vi "SS_Delay_Duration.vi"(6 "Main Cluster IN":T1, 7 "Scan Rate (ms)":i32, 8 "Error In":errorcluster, 11 "Info In":string="\nWaiting for TimerScope Trigger\n- IN: SS TimerScope Trigger\n- OUT: SET SS ThermoRec Received Trigger\nPulse Number is 231123\nPulse Type is 4\n\nDuration (s) is  2.000000\nDelay (s)  is  1.000000\nScan Period (ms) is  15\nNumber of Samples is  134\n\nDelay Started\nDelay Complete\nExternal Measurement of Delay (s): 1.000000\nACQUIRING DATA") -> (0 "Error Out":errorcluster, 3 "Info Out":string="\nWaiting for TimerScope Trigger\n- IN: SS TimerScope Trigger\n- OUT: SET SS ThermoRec Received Trigger\nPulse Number is 231123\nPulse Type is 4\n\nDuration (s) is  2.000000\nDelay (s)  is  1.000000\nScan Period (ms) is  15\nNumber of Samples is  134\n\nDelay Started\nDelay Complete\nExternal Measurement of Delay (s): 1.000000\nACQUIRING DATA", 4 "Main Cluster OUT":T1)   [LabVIEW 2016]
uses:
  Control/Control_Main.ctl
  Control/Control_ModuleArray.ctl
panel:
  in  "Tab Control":enum32{"IN", "OUT", "SubVI Info"}(tab)
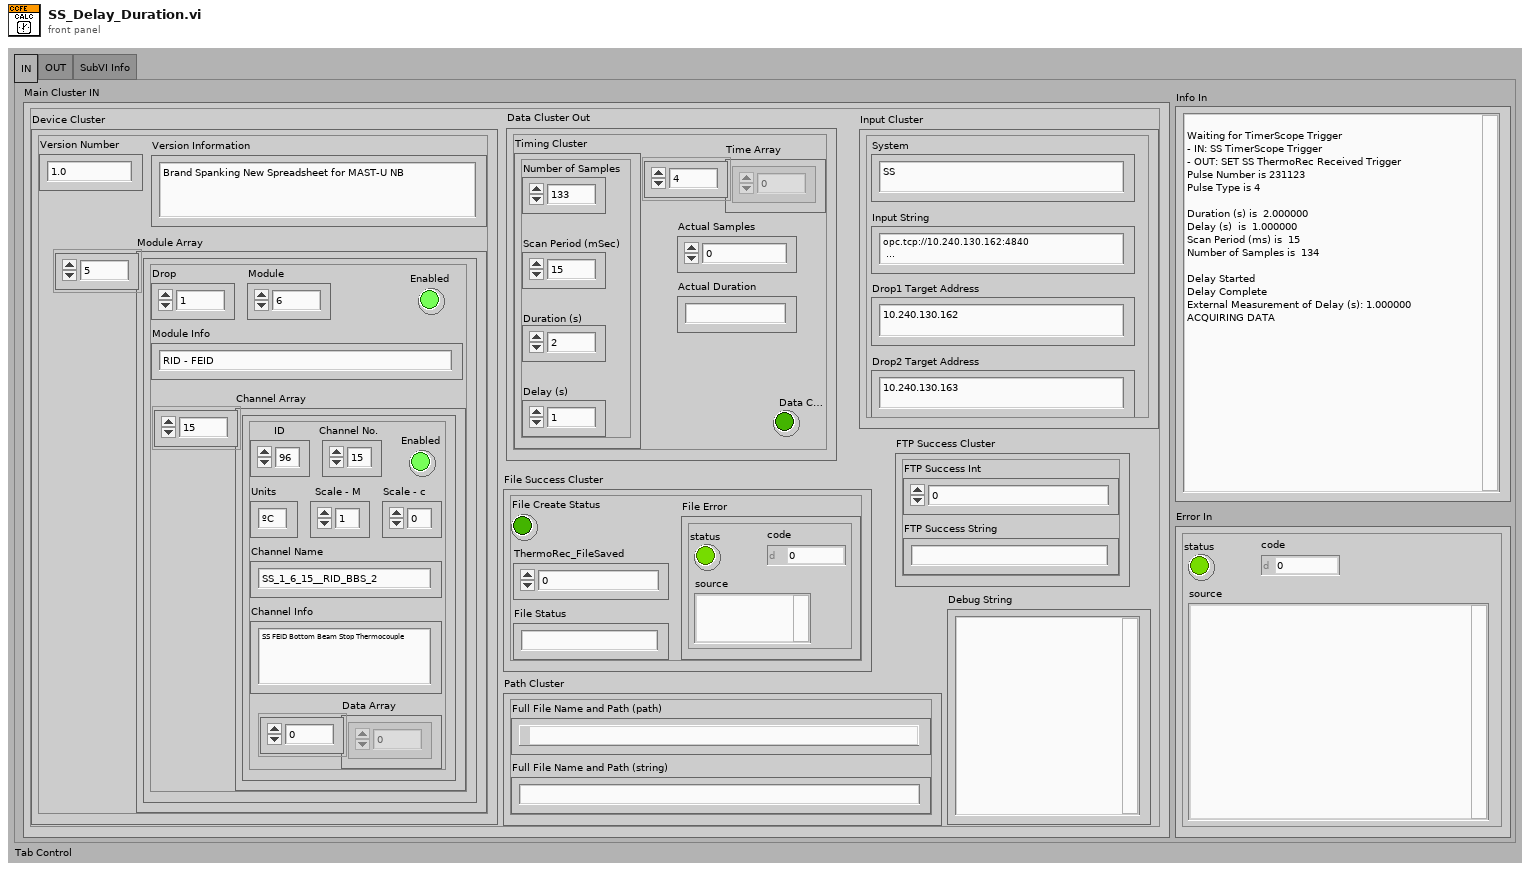
[diagram p1: front panel]
types:
  T1 = typedef "Control_Main.ctl" = cluster{"Device Cluster":cluster{"Module Array":T2, "Version Number":string, "Version Information":string}, "Input Cluster":cluster{"Input String":string, "Drop1 Target Address":string, "Drop2 Target Address":string, "System":string}, "Data Cluster Out":cluster{"Timing Cluster":cluster{"Number of Samples":i32, "Scan Period (mSec)":u32, "Duration (s)":dbl, "Delay (s)":dbl}, "Time Array":dbl[], "Actual Samples":i32, "Actual Duration":string, "Data Collection Error":bool}, "Path Cluster":cluster{"Full File Name and Path (path)":path, "Full File Name and Path (string)":string}, "File Success Cluster":cluster{"ThermoRec_FileSaved":i32, "File Create Status":bool, "File Error":errorcluster, "File Status":string}, "FTP Success Cluster":cluster{"FTP Success Int":i32, "FTP Success String":string}, "Debug String":string}
  T2 = typedef "Control_ModuleArray.ctl" = cluster{"Drop":i32, "Module":i32, "Module Info":string, "Enabled":bool, "Channel Array":cluster{"ID":i32, "Channel No.":i32, "Enabled":bool, "Channel Name":string, "Channel Info":string, "Units":string, "Scale - M":dbl, "Scale - c":dbl, "Data Array":dbl[]}[]}[]
  T3 = cluster{"Number of Samples":i32, "Scan Period (mSec)":u32, "Duration (s)":dbl, "Delay (s)":dbl}
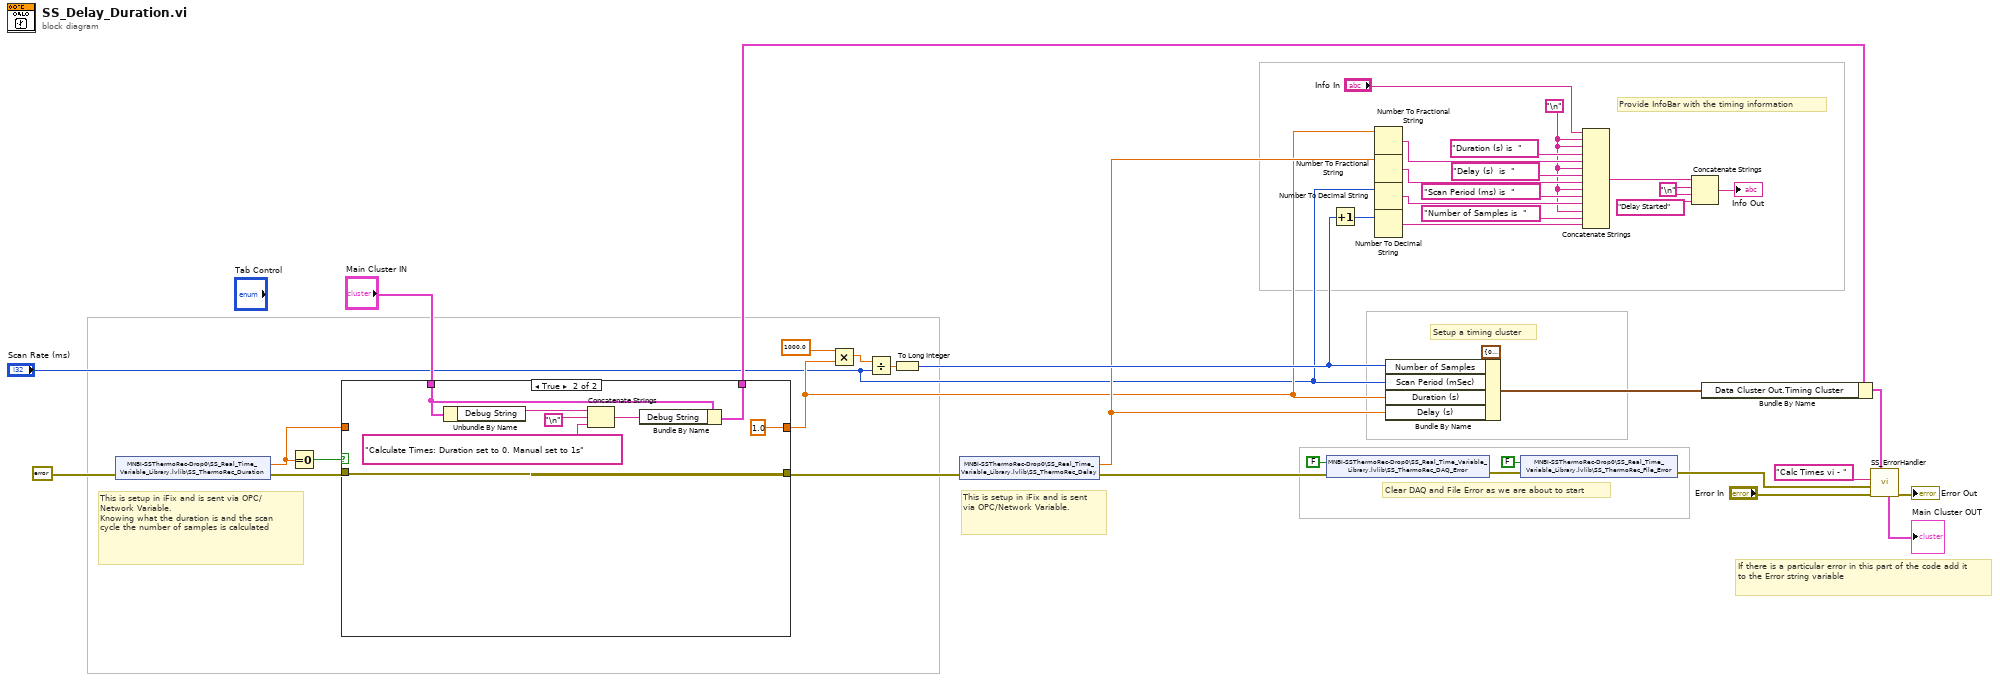
[diagram p0: block diagram]
diagram:
  w27 = "\n"
  w30 = "\n"
  # "This is setup in iFix and is sent via OPC/Network Variable."
  # "If there is a particular error in this part of the code add it to the Error string variable"
  # "Clear DAQ and File Error as we are about to start"
  # "Provide InfoBar with the timing information"
  # "Setup a timing cluster"
  # "This is setup in iFix and is sent via OPC/Network Variable.\nKnowing what the duration is and the scan cycle the number of samples is calculated"
  n1 = shared-variable "MNBI-SSThermoRec-Drop0\\SS_Real_Time_Variable_Library.lvlib\\SS_ThermoRec_Duration"(error in=errorcluster {"status"=FALSE, "code"=0, "source"=""} ("error constant")) -> (w18:dbl, error out=w19:errorcluster)
  n2 = Equal To 0?(x=w18) -> (x = 0?=w20:bool)
  n3 = case shown="True" w20 {
    tunnel: w19 -> [w44 w46]
    tunnel: [w44 w46] -> w16
    tunnel: w18 -> [w43 _]
    tunnel: [w43 1.0 ("y")] -> w7
    tunnel: "Main Cluster IN" -> [w42 w48]
    tunnel: [w42 w49] -> w3
    frame False {
    }
    frame True {
      n4 = Unbundle By Name(w48) -> ("Debug String"=w47:string)
      n5 = Concatenate Strings(w47, "\n", "Calculate Times: Duration set to 0. Manual set to 1s" ("source")) -> (w45:string)
      n6 = Bundle By Name(cluster=w48, "Debug String"=w45) -> (w49:T1)
    }
  }
  n7 = Multiply(x=1000.0, y=w7) -> (x*y=w5:dbl)
  n8 = Divide(x=w5, y="Scan Rate (ms)") -> (x/y=w41:dbl)
  n9 = To Long Integer(number=w41) -> (32bit integer=w32:i32)
  n10 = shared-variable "MNBI-SSThermoRec-Drop0\\SS_Real_Time_Variable_Library.lvlib\\SS_ThermoRec_Delay"(error in=w16) -> (w17:dbl, error out=w15:errorcluster)
  n11 = shared-variable "MNBI-SSThermoRec-Drop0\\SS_Real_Time_Variable_Library.lvlib\\SS_ThermoRec_DAQ_Error"(FALSE ("SS_ThermoRec_DAQ_Error"), error in=w15) -> (error out=w23:errorcluster)
  n12 = Increment(x=w32) -> (x+1=w29:i32)
  n13 = Number To Fractional String(number=w7) -> (F-format string=w39:string)  [unwired: 3 in]
  n14 = Number To Fractional String(number=w17) -> (F-format string=w37:string)  [unwired: 3 in]
  n15 = Number To Decimal String(number="Scan Rate (ms)") -> (decimal integer string=w33:string)  [unwired: 1 in]
  n16 = Number To Decimal String(number=w29) -> (decimal integer string=w31:string)  [unwired: 1 in]
  n17 = Bundle By Name(cluster=T3 {"Number of Samples"=0, "Scan Period (mSec)"=14, "Duration (s)"=0.0, "Delay (s)"=0.0} ("Data Cluster 2"), "Number of Samples"=w32, "Scan Period (mSec)"="Scan Rate (ms)", "Duration (s)"=w7, "Delay (s)"=w17) -> (w22:T3)
  n18 = shared-variable "MNBI-SSThermoRec-Drop0\\SS_Real_Time_Variable_Library.lvlib\\SS_ThermoRec_File_Error"(FALSE ("SS_ThermoRec_DAQ_Error"), error in=w23) -> (error out=w10:errorcluster)
  n19 = Concatenate Strings("Info In", w30, w30, "Duration (s) is  ", w39, w30, "Delay (s)  is  ", w37, w30, "Scan Period (ms) is  ", w33, w30, "Number of Samples is  ", w31) -> (w26:string)
  n20 = Concatenate Strings(w26, w27, w27, "Delay Started") -> (→"Info Out":string)
  n21 = Bundle By Name(cluster=w3, "Data Cluster Out.Timing Cluster"=w22) -> (w9:T1)
  n22 = call "SS_ErrorHandler.vi"("Main Cluster IN"=w9, "Error In"="Error In", "SubVI Error"=w10, "SubVI Name"="Calc Times vi - ") -> ("Error Out"=→"Error Out":errorcluster, "Main Cluster OUT"=→"Main Cluster OUT":T1)  [unwired: 5 in, 1 out]
